vi "module-05-sr-flip-flop.vi"() -> ()   [LabVIEW 2019]
uses:
  samples-common-library/Ctrl_Training_Library_Protected/CtrlTrainingLibary_Protected.lvlib
panel:
  in  "Tab Control":enum32{"Control Panel", "Logic"}(tab)
  in  "Set 1":bool
  in  "Reset 1":bool
  out "Output 1":bool
  out "NOT Output 1":bool
  in  "Set 2":bool
  in  "Reset 2":bool
  out "Ouptut 2":bool
  out "NOT Output 2":bool
  out "Digital State Chart":cluster{dbl, dbl, dbl, dbl, dbl, dbl, dbl, dbl}(graph)
  # "S/R Flip-Flop Test"
  # "Set 1 and Reset 1\nHave edge on\ntriggers"
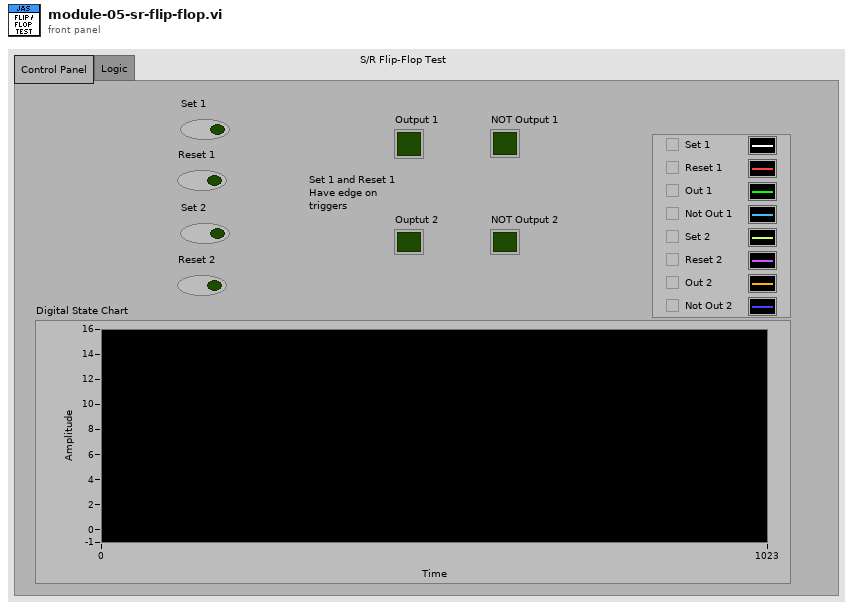
[diagram p1: front panel]
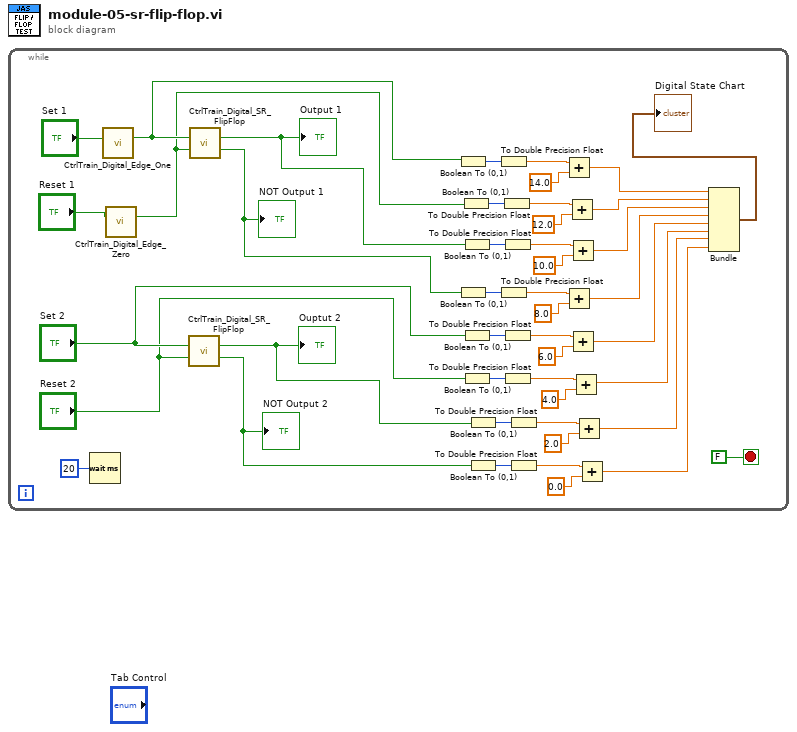
[diagram p0: block diagram]
diagram:
  n1 = while {
    stop <- FALSE stop-if-true
    n2 = Wait (ms)(milliseconds to wait=u32 20) -> ()  [unwired: 1 out]
    n3 = call "CtrlTrain_Digital_Edge_One.vi"("Input"="Set 1") -> ("Output"=w8:bool)  [unwired: 14 in]
    n4 = call "CtrlTrain_Digital_Edge_Zero.vi"("Input"="Reset 1") -> ("Output"=w7:bool)  [unwired: 14 in]
    n5 = call "CtrlTrain_Digital_SR_FlipFlop.vi"("Set"="Set 2", "Reset"="Reset 2") -> ("Output"=w2:bool, "Inverse Output"=w1:bool)  [unwired: 12 in]
    "Ouptut 2" <- w2
    "NOT Output 2" <- w1
    n6 = call "CtrlTrain_Digital_SR_FlipFlop.vi"("Set"=w8, "Reset"=w7) -> ("Output"=w6:bool, "Inverse Output"=w5:bool)  [unwired: 12 in]
    "Output 1" <- w6
    "NOT Output 1" <- w5
    n7 = Boolean To (0,1)(Boolean=w8) -> (0, 1=w24:i16)
    n8 = Boolean To (0,1)(Boolean=w5) -> (0, 1=w25:i16)
    n9 = Boolean To (0,1)(Boolean=w7) -> (0, 1=w27:i16)
    n10 = Boolean To (0,1)(Boolean=w6) -> (0, 1=w29:i16)
    n11 = Boolean To (0,1)(Boolean="Set 2") -> (0, 1=w31:i16)
    n12 = Boolean To (0,1)(Boolean="Reset 2") -> (0, 1=w33:i16)
    n13 = Boolean To (0,1)(Boolean=w2) -> (0, 1=w13:i16)
    n14 = Boolean To (0,1)(Boolean=w1) -> (0, 1=w15:i16)
    n15 = To Double Precision Float(number=w24) -> (double precision float=w40:dbl)
    n16 = To Double Precision Float(number=w25) -> (double precision float=w26:dbl)
    n17 = To Double Precision Float(number=w27) -> (double precision float=w28:dbl)
    n18 = To Double Precision Float(number=w29) -> (double precision float=w30:dbl)
    n19 = To Double Precision Float(number=w31) -> (double precision float=w32:dbl)
    n20 = To Double Precision Float(number=w33) -> (double precision float=w34:dbl)
    n21 = To Double Precision Float(number=w13) -> (double precision float=w14:dbl)
    n22 = To Double Precision Float(number=w15) -> (double precision float=w16:dbl)
    n23 = Add(x=w40, y=14.0) -> (x+y=w41:dbl)
    n24 = Add(x=w26, y=8.0) -> (x+y=w39:dbl)
    n25 = Add(x=w28, y=12.0) -> (x+y=w37:dbl)
    n26 = Add(x=w30, y=10.0) -> (x+y=w38:dbl)
    n27 = Add(x=w32, y=6.0) -> (x+y=w35:dbl)
    n28 = Add(x=w34, y=4.0) -> (x+y=w36:dbl)
    n29 = Add(x=w14, y=2.0) -> (x+y=w10:dbl)
    n30 = Add(x=w16, y=0.0) -> (x+y=w9:dbl)
    n31 = Bundle(w41, w37, w38, w39, w35, w36, w10, w9) -> (→"Digital State Chart":cluster{dbl, dbl, dbl, dbl, dbl, dbl, dbl, dbl})  [unwired: 1 in]
  }
